vi "Current Controller.vi"() -> ()   [LabVIEW 2015]
uses:
  <vilib>/rvi/Emulation/niFpgaGetClockAttributes.vi
  <vilib>/rvi/Emulation/niFpgaSctlEmulationGetInTimedLoop.vi
  <vilib>/rvi/Emulation/niFpgaEmulationReportErrorSimple.vi
  <vilib>/rvi/eio/common/nirviEmuTemplateMethod_errors.vi
  <vilib>/rvi/interface/RandomDataEmulation/niFpgaRandomDataHandleErrors.vi
  <vilib>/rvi/Emulation/niFpgaCriticalErrorInLSC.vi
  <vilib>/eio/EIONode/EIONode.xnode
  <vilib>/rvi/DataTransferAndStorage/Container/XNode/niFpgaContainer.xnode
  <vilib>/rvi/interface/RandomDataEmulation/nirviRandomDataFpgaReadWriteTemplate.vi
panel:
  in  "Outlet Count(uSec)":i32=500000 caption="Count(uSec)"
  out "Outlet Overflow?":bool
  in  "DAC Outlet Valve":i32(knob)=323 min=0 max=400 scale=0.0..400.0 scale format="%.2f"
  in  "Inlet Count(uSec)":i32=500000 caption="Count(uSec)"
  out "Inlet Overflow?":bool
  in  "DAC Inlet Valve":i32(knob)=323 min=0 max=400 scale=0.0..400.0 scale format="%.2f"
  # "Overview.\n\nThis demonstrates how to control the PVQ-33-16-5G proportional solenoid valve. Wire the AO0 pin on the C connector of the myRIo to the pin 3 of the non-inverting input of the opamp. Connect the power supplies and follow these instructions:\n\nInstructions:\n1.        Operate at constant pressure of 30 psi to get best results\n2.        Operate this valve between the DAC resolutions of 240 and  394 only. If you operate outside of this range, you might damage the valve.\n3.        Run the VI."
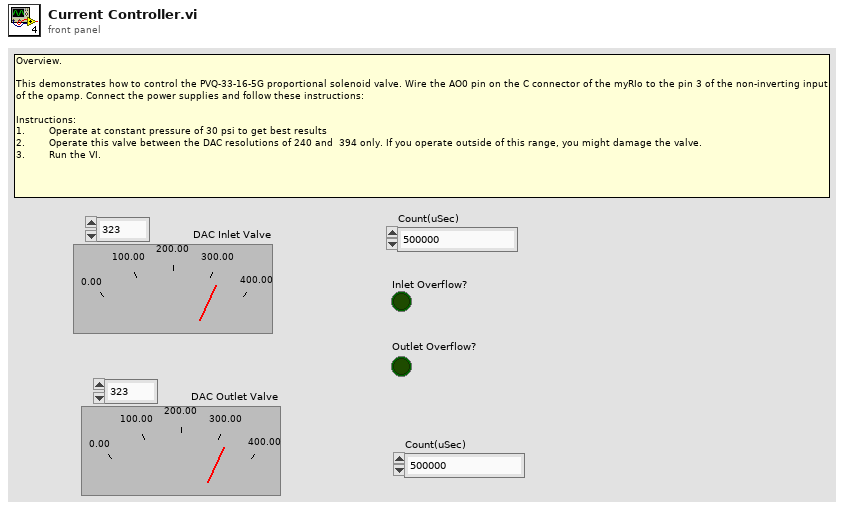
[diagram p1: front panel]
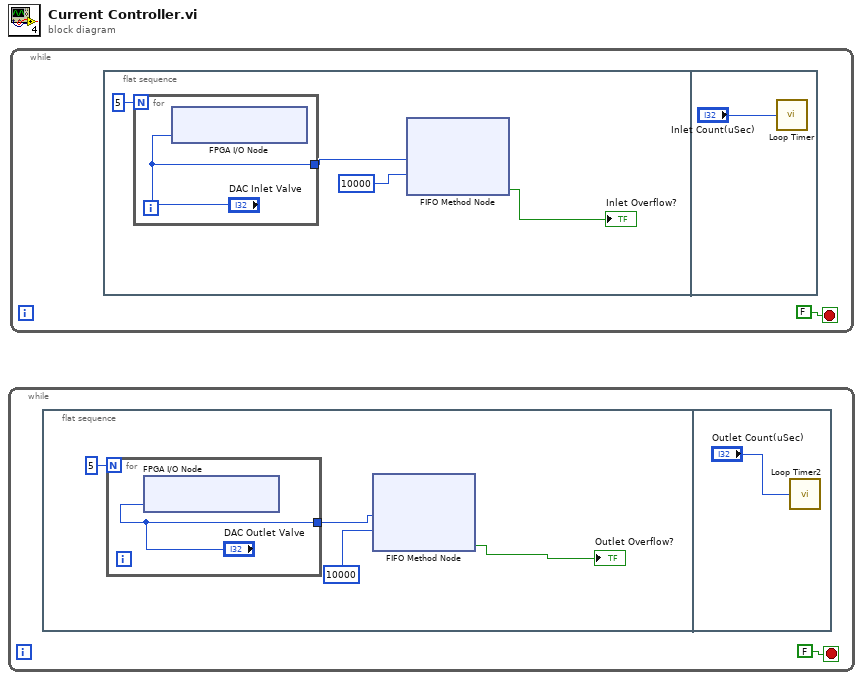
[diagram p0: block diagram]
diagram:
  n1 = while {
    stop <- FALSE stop-if-true
    n2 = flat-sequence {
      frame #0 {
        n3 = for {
          N: 5 -> [_]
          tunnel: ["DAC Outlet Valve"] -> w4
          n4 = xnode "FPGA I/O Node"("ConnectorC/AO1"="DAC Outlet Valve") -> ()  [unwired: 1 in, 1 out]
        }
        n5 = xnode ("FIFO Method Node")("Element"=w4, "Timeout"=10000) -> ("Timed Out?"=→"Outlet Overflow?":bool)  [unwired: 1 in, 1 out]
      }
      frame #1 {
        n6 = call "Loop Timer2"("Count(uSec)"="Outlet Count(uSec)") -> ()  [unwired: 1 out]
      }
    }
  }
  n7 = while {
    stop <- FALSE stop-if-true
    n8 = flat-sequence {
      frame #0 {
        n9 = for {
          N: 5 -> [_]
          tunnel: ["DAC Inlet Valve"] -> w12
          n10 = xnode "FPGA I/O Node"("ConnectorC/AO0"="DAC Inlet Valve") -> ()  [unwired: 1 in, 1 out]
        }
        n11 = xnode ("FIFO Method Node")("Element"=w12, "Timeout"=10000) -> ("Timed Out?"=→"Inlet Overflow?":bool)  [unwired: 1 in, 1 out]
      }
      frame #1 {
        n12 = call "Loop Timer"("Count(uSec)"="Inlet Count(uSec)") -> ()  [unwired: 1 out]
      }
    }
  }
